vi "FGV Variant DB.vi"(9 "Data":variant, 10 "name":string, 11 "Enum":enum16{"Set Data", "Reset Data", "Get Data"}(ring)) -> (1 "found?":bool, 2 "replaced?":bool, 3 "Value":variant)   [LabVIEW 2019]
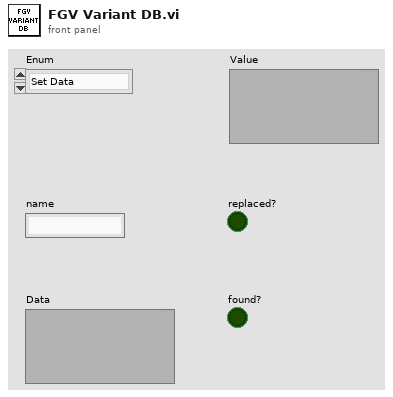
[diagram p1: front panel]
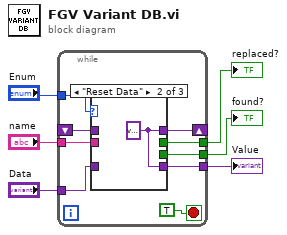
[diagram p0: block diagram]
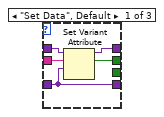
[diagram p2: hidden frame]
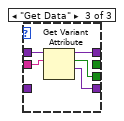
[diagram p3: hidden frame]
diagram:
  n1 = while {
    tunnel: "Enum" -> [w14]
    shift-right: [w13] -> _
    shift-left: _ -> [w12]
    tunnel: "name" -> [w11]
    tunnel: "Data" -> [w10]
    tunnel: [w9] -> w3
    tunnel: [w8] -> w2
    tunnel: [w7] -> w1
    stop <- TRUE stop-if-true
    n2 = case shown="\"Reset Data\"" w14 {
      tunnel: [w18 w21 w24] -> w13
      tunnel: w12 -> [w20 _ w26]
      tunnel: w11 -> [w19 _ w25]
      tunnel: w10 -> [w16 _ _]
      tunnel: [w17 _ _] -> w9
      tunnel: [_ _ w23] -> w8
      tunnel: [w16 w21 w22] -> w7
      frame "Set Data", Default {
        n3 = Set Variant Attribute(Variant=w20, name=w19, value=w16) -> (Variant out=w18:variant, replaced=w17:bool)  [unwired: 1 in, 1 out]
      }
      frame "Reset Data" {
        w21 = variant
      }
      frame "Get Data" {
        n4 = Get Variant Attribute(Variant=w26, name=w25) -> (duplicate Variant=w24:variant, found=w23:bool, value=w22:variant)  [unwired: 2 in, 1 out]
      }
    }
  }
  "replaced?" <- w3
  "found?" <- w2
  "Value" <- w1
